vi "2dInterpol.vi"(6 "empty image":bool, 8 "final":T1, 11 "Z":dbl[][](graph)) -> (0 "Sum Y":cluster{"Ramp Pattern":dbl[], dbl[]}, 1 "spec cluster 2":cluster{"Momentum [MeV/C]":dbl[], dbl[]}(graph), 3 "charge density":dbl[][](array[numeric]), 5 "time: 2Dinter":u32)   [LabVIEW 2013]
uses:
  finalCalibTypdef.ctl
  <vilib>/Analysis/8numeric.llb/1D Numeric Integration.vi
  <vilib>/gmath/interp.llb/Interpolate 2D (2d X,Y).vi
  <vilib>/Analysis/NI_AALPro.lvlib
  <vilib>/gmath/NI_Gmath.lvlib
panel:
  out "charge (sum)":dbl
  out "Array":dbl[][](array[numeric])
  out "time: spectra":u32
  out "time: prepare arrays":u32
  out "charge (YSum)":dbl format="%0.4f"
  out "charge (spectra)":dbl format="%0.4f"
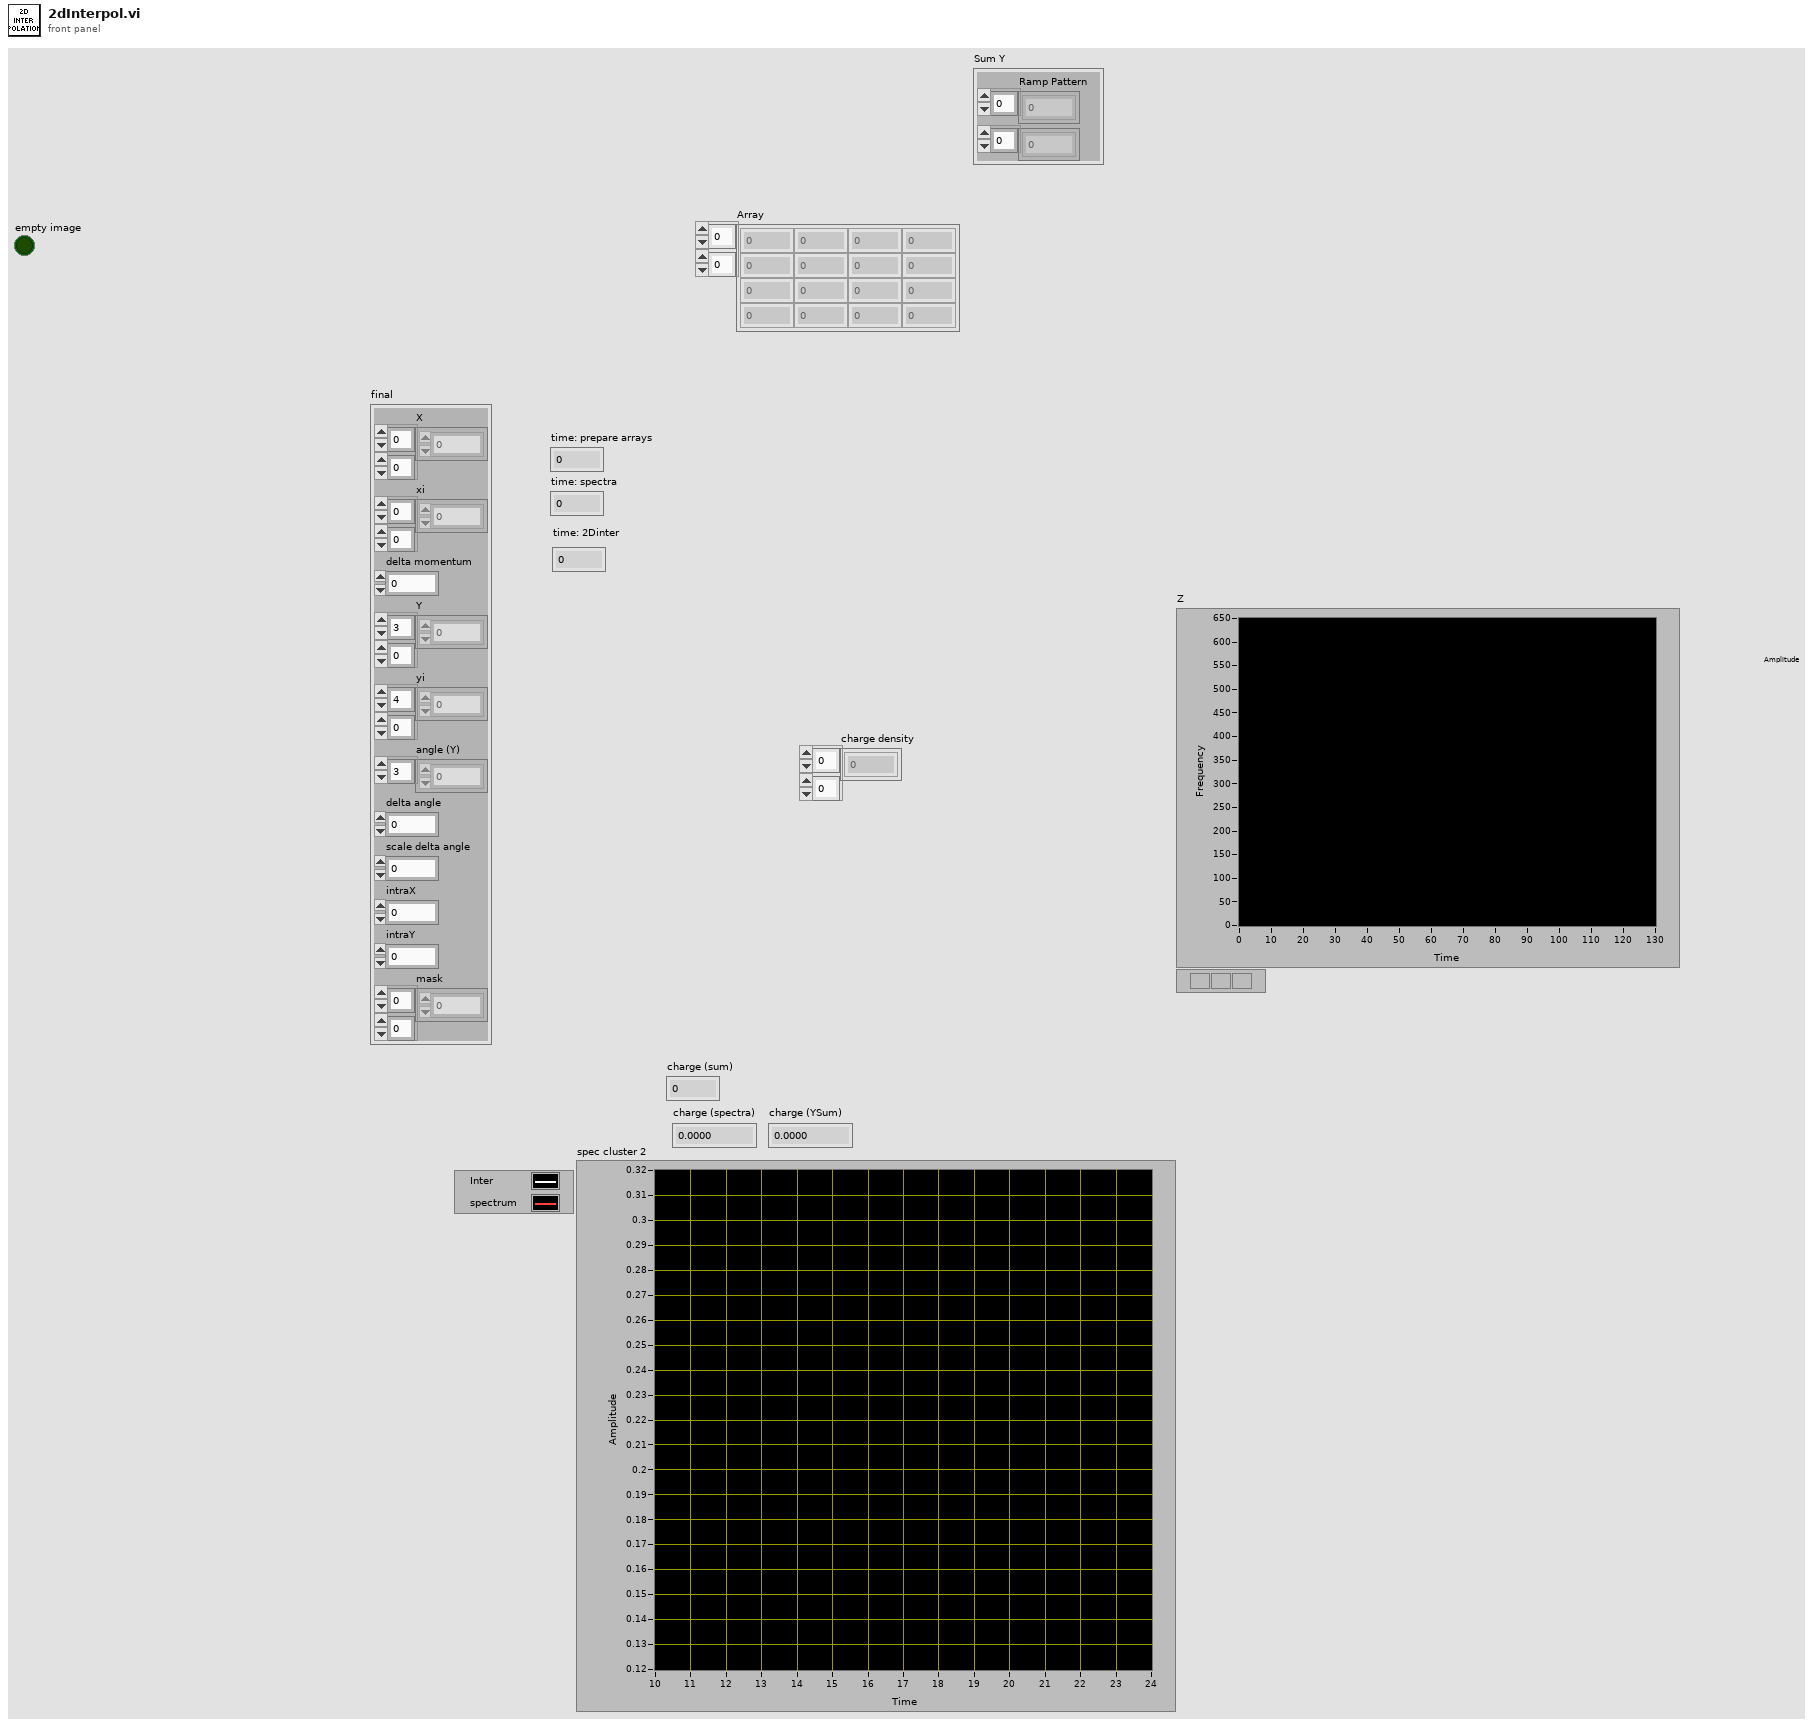
[diagram p1: front panel]
types:
  T1 = typedef "finalCalibTypdef.ctl" = cluster{"X":dbl[][], "xi":dbl[][], "delta momentum":dbl, "Y":dbl[][], "yi":dbl[][], "angle (Y)":dbl[], "delta angle":dbl, "scale delta angle":dbl, "intraX":dbl, "intraY":dbl, "mask":dbl[][]}
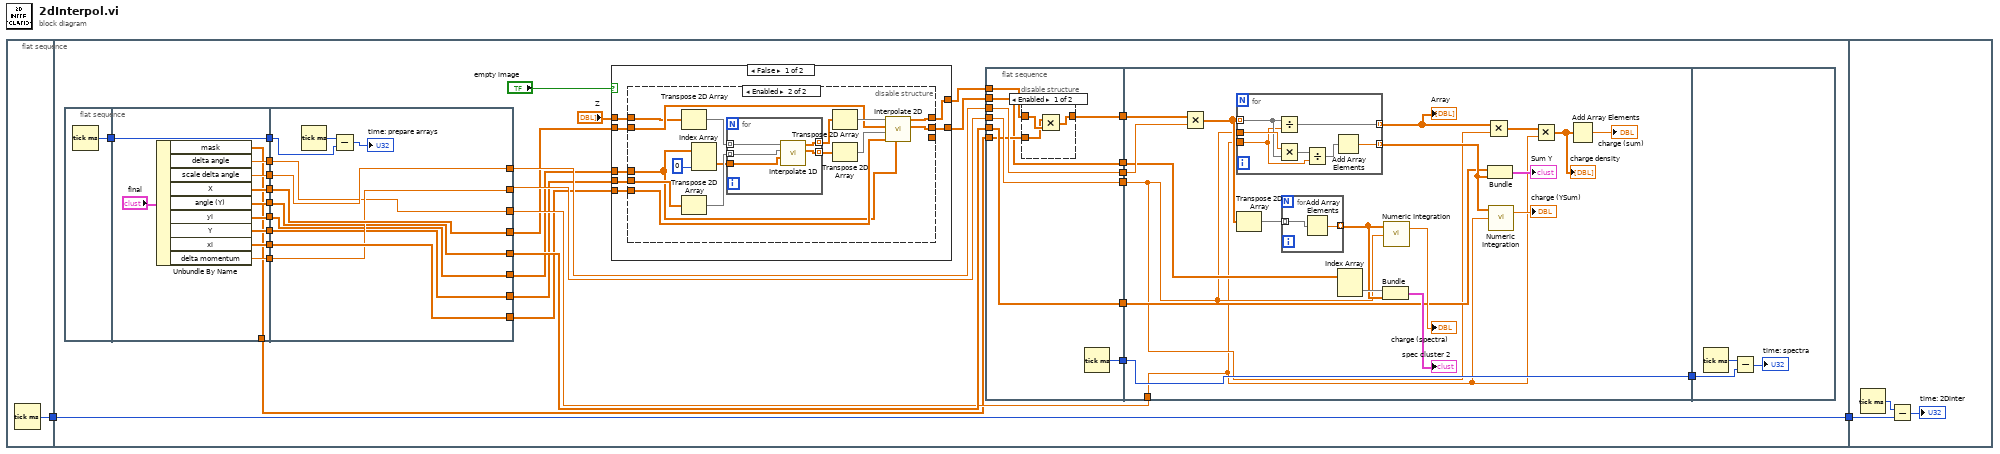
[diagram p0: block diagram]
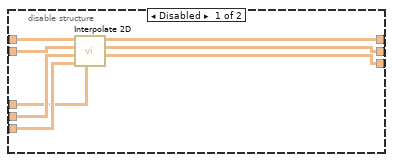
[diagram p2: hidden frame]
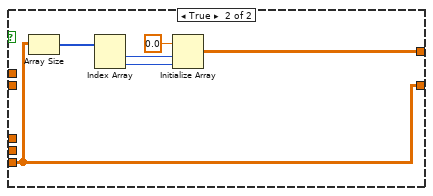
[diagram p3: hidden frame]
diagram:
  n1 = flat-sequence {
    tunnel: [w3] -> w2
    tunnel: w2 -> [w34]
    tunnel: [w34] -> w1
    tunnel: w1 -> [w145]
    frame #0 {
      n2 = Tick Count (ms)() -> (millisecond timer value=w3:u32)
    }
    frame #1 {
      n3 = flat-sequence {
        tunnel: [w121] -> w22
        tunnel: [w132] -> w29
        tunnel: [w131] -> w28
        tunnel: [w130] -> w27
        tunnel: [w124] -> w26
        tunnel: [w129] -> w25
        tunnel: [w128] -> w24
        tunnel: [w127] -> w23
        tunnel: w22 -> [w126]
        tunnel: [w126] -> w21
        tunnel: [w125] -> w11
        tunnel: [w123] -> w4
        tunnel: [w138] -> w7
        tunnel: [w139] -> w6
        tunnel: [w140] -> w30
        tunnel: [w134] -> w32
        tunnel: [w141] -> w13
        tunnel: [w142] -> w5
        tunnel: [w143] -> w8
        tunnel: w29 -> [w143]
        tunnel: w28 -> [w142]
        tunnel: w27 -> [w141]
        tunnel: w26 -> [w134]
        tunnel: w25 -> [w140]
        tunnel: w24 -> [w139]
        tunnel: w23 -> [w138]
        tunnel: w21 -> [w136]
        tunnel: [w133] -> w10
        tunnel: w11 -> [w133]
        frame #0 {
          n4 = Tick Count (ms)() -> (millisecond timer value=w121:u32)
        }
        frame #1 {
          n5 = Unbundle By Name("final") -> ("mask"=w123:dbl[][], "delta angle"=w125:dbl, "scale delta angle"=w129:dbl, "X"=w132:dbl[][], "angle (Y)"=w124:dbl[], "yi"=w127:dbl[][], "Y"=w128:dbl[][], "xi"=w131:dbl[][], "delta momentum"=w130:dbl)
        }
        frame #2 {
          n6 = Tick Count (ms)() -> (millisecond timer value=w137:u32)
          n7 = Subtract(x=w137, y=w136) -> (x-y=→"time: prepare arrays":u32)
        }
      }
      n8 = case shown="False" "empty image" {
        tunnel: w8 -> [w38 _]
        tunnel: [w35 w75] -> w33
        tunnel: w5 -> [w37 w75]
        tunnel: "Z" -> [w41 _]
        tunnel: [w36 w71] -> w31
        tunnel: w6 -> [w40 _]
        tunnel: w7 -> [w39 _]
        frame False {
          n9 = disable-structure shown="Enabled" {
            disable-tunnel: w38 -> [w50 w61]
            disable-tunnel: [w49 w58] -> w35
            disable-tunnel: w37 -> [w48 w60]
            disable-tunnel: w41 -> [w47 w57]
            disable-tunnel: [w46 w59] -> w36
            disable-tunnel: w40 -> [w45 w54]
            disable-tunnel: [w43 _] -> _
            disable-tunnel: w39 -> [w42 w52]
            frame Disabled {
              n10 = call-poly <vilib>:"Interpolate 2D.vi"("yi"=w42, "xi"=w48, "Y"=w45, "X"=w50, "Z"=w47) -> ("error"=w44:i32, "yi used"=w43:dbl[][], "xi used"=w49:dbl[][], "zi"=w46:dbl[][])  [unwired: 3 in]
            }
            frame Enabled {
              n11 = Transpose 2D Array(2D array=w57) -> (transposed array=w55:dbl[][])
              n12 = Transpose 2D Array(2D array=w54) -> (transposed array=w53:dbl[][])
              n13 = Index Array(array=w52, index (col)=0 ("disabled index (col)")) -> (element=w51:dbl[])  [unwired: 1 in]
              n14 = for {
                tunnel: w55 -> [w70] mode=indexing
                tunnel: w53 -> [w69] mode=indexing
                tunnel: w51 -> [w68]
                tunnel: [w67] -> w65 mode=indexing
                tunnel: [w66] -> w63 mode=indexing
                n15 = call <vilib>:"Interpolate 1D.vi"("xi"=w68, "X"=w69, "Y"=w70) -> ("xi used"=w66:dbl[], "yi"=w67:dbl[])  [unwired: 6 in, 1 out]
              }
              n16 = Transpose 2D Array(2D array=w65) -> (transposed array=w64:dbl[][])
              n17 = Transpose 2D Array(2D array=w63) -> (transposed array=w62:dbl[][])
              n18 = call-poly <vilib>:"Interpolate 2D.vi"("yi"=w52, "xi"=w60, "Y"=w62, "X"=w61, "Z"=w64) -> ("xi used"=w58:dbl[][], "zi"=w59:dbl[][])  [unwired: 3 in, 2 out]
            }
          }
        }
        frame True {
          n19 = Array Size(array=w75) -> (size(s)=w74:i32[])
          n20 = Index Array(array=w74) -> (element #1=w73:i32, element #2=w72:i32)  [unwired: 2 in]
          n21 = Initialize Array(0.0 ("element"), w73, w72) -> (w71:dbl[][])
        }
      }
      n22 = flat-sequence {
        tunnel: w30 -> [w83]
        tunnel: w31 -> [w80]
        tunnel: w32 -> [w84]
        tunnel: w33 -> [w77]
        tunnel: [w77] -> w20
        tunnel: [w84] -> w19
        tunnel: [w78] -> w18
        tunnel: [w83] -> w17
        tunnel: [w82] -> w16
        tunnel: w13 -> [w81]
        tunnel: [w81] -> w12
        tunnel: w4 -> [w79]
        tunnel: w10 -> [w91]
        tunnel: w20 -> [w96]
        tunnel: w19 -> [w101]
        tunnel: w18 -> [w99]
        tunnel: w17 -> [w98]
        tunnel: w16 -> [w97]
        tunnel: [w97] -> w15
        tunnel: w12 -> [w93]
        tunnel: w15 -> [w119]
        frame #0 {
          n23 = disable-structure shown="Enabled" {
            disable-tunnel: w80 -> [w87 w88]
            disable-tunnel: w79 -> [w86 _]
            disable-tunnel: [w85 w88] -> w78
            frame Enabled {
              n24 = Multiply(x=w86, y=w87) -> (x*y=w85:dbl[][])
            }
            frame Disabled {
            }
          }
          n25 = Tick Count (ms)() -> (millisecond timer value=w82:u32)
        }
        frame #1 {
          n26 = Multiply(x=w99, y=w98) -> (x*y=w95:dbl[][])
          n27 = for {
            tunnel: w95 -> [w113] mode=indexing
            tunnel: [w117] -> w102 mode=indexing
            tunnel: w93 -> [w114]
            tunnel: w91 -> [w112]
            tunnel: [w111] -> w94 mode=indexing
            n28 = Divide(x=w113, y=w112) -> (x/y=w111:dbl[])
            n29 = Multiply(x=w114, y=w113) -> (x*y=w116:dbl[])
            n30 = Divide(x=w116, y=w112) -> (x/y=w115:dbl[])
            n31 = Add Array Elements(numeric array=w115) -> (sum=w117:dbl)
          }
          "Array" <- w94
          n32 = Transpose 2D Array(2D array=w95) -> (transposed array=w108:dbl[][])
          n33 = for {
            tunnel: w108 -> [w109] mode=indexing
            tunnel: [w110] -> w105 mode=indexing
            n34 = Add Array Elements(numeric array=w109) -> (sum=w110:dbl)
          }
          n35 = Index Array(array=w96) -> (element=w106:dbl[])  [unwired: 2 in]
          n36 = Bundle("xi"=w106, w105) -> (→"spec cluster 2":cluster{"xi":dbl[], dbl[]})  [unwired: 1 in]
          n37 = call-poly <vilib>:"Numeric Integration.vi"("dt"=w93, "Input Array"=w105) -> ("result"=→"charge (spectra)":dbl)  [unwired: 1 in, 1 out]
          n38 = Multiply(x=w94, y=w93) -> (x*y=w92:dbl[][])
          n39 = Bundle("angle (Y)"=w101, w102) -> (→"Sum Y":cluster{"angle (Y)":dbl[], dbl[]})  [unwired: 1 in]
          n40 = call-poly <vilib>:"Numeric Integration.vi"("dt"=w91, "Input Array"=w102) -> ("result"=→"charge (YSum)":dbl)  [unwired: 1 in, 1 out]
          n41 = Multiply(x=w92, y=w91) -> (x*y=w90:dbl[][])
          "charge density" <- w90
          n42 = Add Array Elements(numeric array=w90) -> (sum=→"charge (sum)":dbl)
        }
        frame #2 {
          n43 = Tick Count (ms)() -> (millisecond timer value=w120:u32)
          n44 = Subtract(x=w120, y=w119) -> (x-y=→"time: spectra":u32)
        }
      }
    }
    frame #2 {
      n45 = Tick Count (ms)() -> (millisecond timer value=w146:u32)
      n46 = Subtract(x=w146, y=w145) -> (x-y=→"time: 2Dinter":u32)
    }
  }
